vi "MALT24VI set one output.vi"() -> ()   [LabVIEW 2018]
uses:
  <instrlib>/AltonTech MALT/AltonTech MALT200817.lvlib
panel:
  in  "Yn":i32=1
  in  "Address":i32=3 format="%02x"
  in  "Y1":bool
  in  "stop":bool
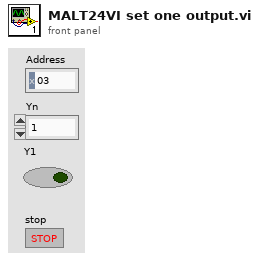
[diagram p1: front panel]
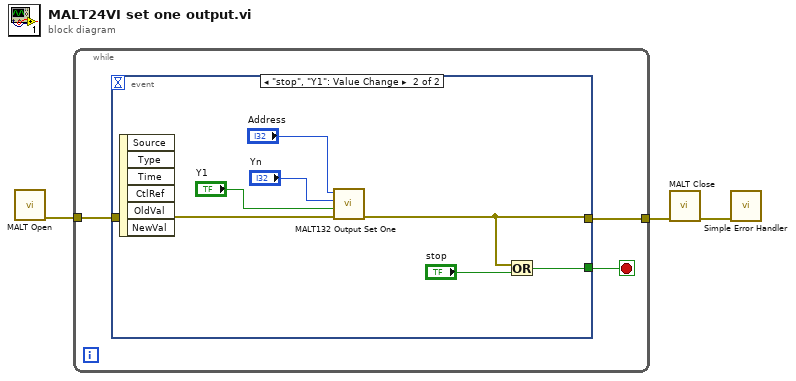
[diagram p0: block diagram]
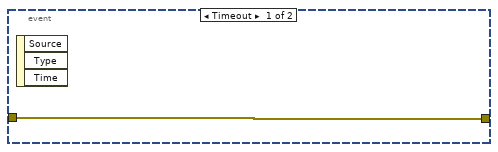
[diagram p2: hidden frame]
diagram:
  n1 = call <instrlib>:"MALT Open.vi"() -> ("error out"=w3:errorcluster)  [unwired: 10 in, 1 out]
  n2 = while {
    tunnel: w3 -> [w6]
    tunnel: [w5] -> w2
    stop <- w4 stop-if-true
    n3 = event shown="[1] \"stop\", \"Y1\": Value Change" {
      selector: _ -> [_ _]
      dyn-events: _ -> [_ _]
      timeout: _ -> [_ _]
      tunnel: w6 -> [w7 w13]
      tunnel: [w7 w12] -> w5
      tunnel: [_ w10] -> w4
      event Timeout {
        n4 = event-data() -> ()  [unwired: 1 in, 3 out]
      }
      event "stop", "Y1": Value Change {
        n5 = event-data() -> ()  [unwired: 1 in, 6 out]
        n6 = call <instrlib>:"MALT132 Output Set One.vi"("error in"=w13, "State"="Y1", "Kn"="Yn", "Address"="Address") -> ("error out"=w12:errorcluster)  [unwired: 7 in]
        n7 = Or(x=w12, y="stop") -> (x .or. y?=w10:bool)
      }
    }
  }
  n8 = call <instrlib>:"MALT Close.vi"("error in"=w2) -> ("error out"=w1:errorcluster)  [unwired: 10 in]
  n9 = call <vilib>:"Simple Error Handler.vi"("error in (no error)"=w1) -> ()  [unwired: 4 in, 5 out]
